vi "sv_Check for Weighting Conflict.vi"(6 "weighting":T1 items=["Linear", "A-weighting", "B-weighting", "C-weighting", "ITU-R 468-4", "Dolby", "CCITT", "C-message", "Wb", "Wc", "Wd", "We", "Wf", "Wh", "Wj", "Wk", "Wm", "AES17 20 kHz lowpass", "AES17 40 kHz lowpass", "AES17 20 kHz highpass", "AES17 40 kHz highpass"], 8 "error in (no error)":errorcluster, 11 "scaled signal [EU]":waveform(dbl)) -> (0 "error out":errorcluster, 3 "scaled signal [EU]":waveform(dbl), 4 "dup weighting":T1 items=["Linear", "A-weighting", "B-weighting", "C-weighting", "ITU-R 468-4", "Dolby", "CCITT", "C-message", "Wb", "Wc", "Wd", "We", "Wf", "Wh", "Wj", "Wk", "Wm", "AES17 20 kHz lowpass", "AES17 40 kHz lowpass", "AES17 20 kHz highpass", "AES17 40 kHz highpass"])   [LabVIEW 2017]
doc: "Make sure we will not be applying weighting twice if an external weighting filter has been used"
uses:
  <vilib>/addons/_NISVFA/_Shared subVIs/Controls/svc_Weighting Filter Text Ring.ctl
  <vilib>/addons/_NISVFA/_Shared subVIs/Common/svc_Set SV Channel Info (variant).vi
  <vilib>/addons/_NISVFA/_Shared subVIs/Common/SVL Set dB Reference (variant).vi
  <vilib>/addons/_NISVFA/_Shared subVIs/Common/svc_Engineering Units to Unit Label.vi
  <vilib>/addons/_NISVFA/_Shared subVIs/Common/svc_Unit Label to Engineering Units.vi
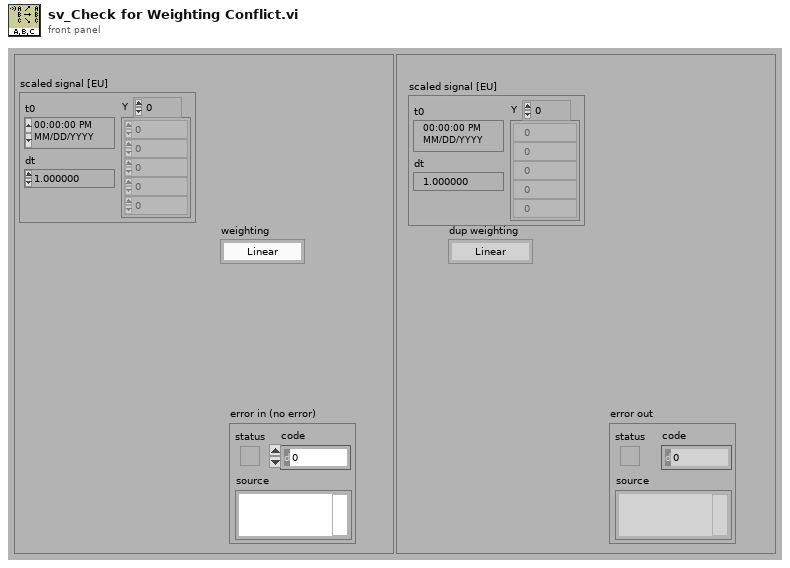
[diagram p1: front panel]
types:
  T1 = typedef "svc_Weighting Filter Text Ring.ctl" = u16
  T2 = typedef "svc_Channel Info.ctl" = cluster{"sensor sensitivity":dbl, "engineering units":T3, "dB reference":dbl, "custom label":string, "weighting filter":T1, "pregain":dbl}
  T3 = typedef "svc_Engineering Units Text Ring.ctl" = u16
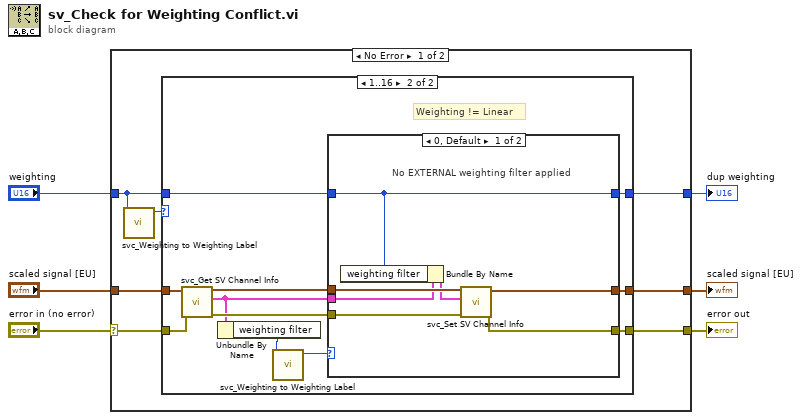
[diagram p0: block diagram]
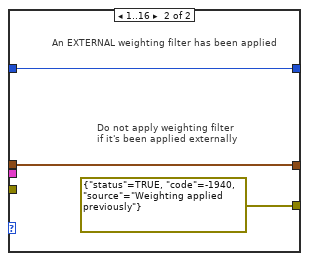
[diagram p3: hidden frame]
diagram:
  n1 = case shown="No Error" "error in (no error)" {
    selector: "error in (no error)" -> [w13 w40]
    tunnel: "weighting" -> [w9 w38]
    tunnel: [w7 w40] -> w5
    tunnel: [w8 w38] -> w4
    tunnel: "scaled signal [EU]" -> [w12 w39]
    tunnel: [w11 w39] -> w1
    frame No Error {
      n2 = call <vilib>:"svc_Weighting to Weighting Label.vi"("weighting filter"=w9) -> ("weighting enum"=w10:T1)  [unwired: 9 in, 1 out]
      n3 = case shown="1..16" w10 {
        tunnel: [w16 w25] -> w8
        tunnel: w13 -> [w14 w24]
        tunnel: [w14 w27] -> w7
        tunnel: w12 -> [w15 w23]
        tunnel: [w15 w26] -> w11
        tunnel: w9 -> [w16 w19]
        frame 0, Default {
          # "Weighting = Linear...\ndo nothing"
        }
        frame 1..16 {
          # "Weighting != Linear"
          n4 = call <vilib>:"svc_Get SV Channel Info.vi"("error in (no error)"=w24, "scaled signal [EU]"=w23) -> ("error out"=w21:errorcluster, "channel info"=w20:T2, "dup scaled signal [EU]"=w22:waveform(dbl))  [unwired: 4 in, 3 out]
          n5 = Unbundle By Name(w20) -> ("weighting filter"=w18:T1)
          n6 = call <vilib>:"svc_Weighting to Weighting Label.vi"("weighting filter"=w18) -> ("weighting enum"=w17:T1)  [unwired: 9 in, 1 out]
          n7 = case shown="0, Default" w17 {
            tunnel: [w33 errorcluster {"status"=TRUE, "code"=-1940, "source"="Weighting applied previously"} ("error out")] -> w27
            tunnel: [w34 w37] -> w26
            tunnel: w21 -> [w32 _]
            tunnel: w22 -> [w31 w37]
            tunnel: w19 -> [w30 w35]
            tunnel: [w30 w35] -> w25
            tunnel: w20 -> [w29 _]
            frame 0, Default {
              # "No EXTERNAL weighting filter applied"
              n8 = Bundle By Name(cluster=w29, "weighting filter"=w30) -> (w28:T2)
              n9 = call <vilib>:"svc_Set SV Channel Info.vi"("error in (no error)"=w32, "channel info"=w28, "scaled signal in"=w31) -> ("error out"=w33:errorcluster, "scaled signal out"=w34:waveform(dbl))  [unwired: 7 in]
            }
            frame 1..16 {
              # "Do not apply weighting filter\nif it's been applied externally"
              # "An EXTERNAL weighting filter has been applied"
            }
          }
        }
      }
    }
    frame Error {
    }
  }
  "dup weighting" <- w4
  "error out" <- w5
  "scaled signal [EU]" <- w1
